vi "StateMachineExecute.vi"(5 "States finished?":bool=TRUE, 8 "error in (no error)":errorcluster, 11 "StateMachine in":refnum<class "StateMachine.lvclass">) -> (0 "error out":errorcluster, 2 "output cluster":T1, 3 "StateMachine out":refnum<class "StateMachine.lvclass">)   [LabVIEW 2018, in "StateMachine.lvclass"]
uses:
  StateMachine.lvclass
  StateMachine.lvclass/StateMachine.ctl
  <vilib>/Rock Robotics/WPI/ThirdParty/Phoenix-LabVIEW/Motor Controller/Controls/CTRE_Phoenix_MotorControl_ControlMode.ctl
  <vilib>/Rock Robotics/WPI/Solenoid/WPI_SolenoidSetEnum.vi
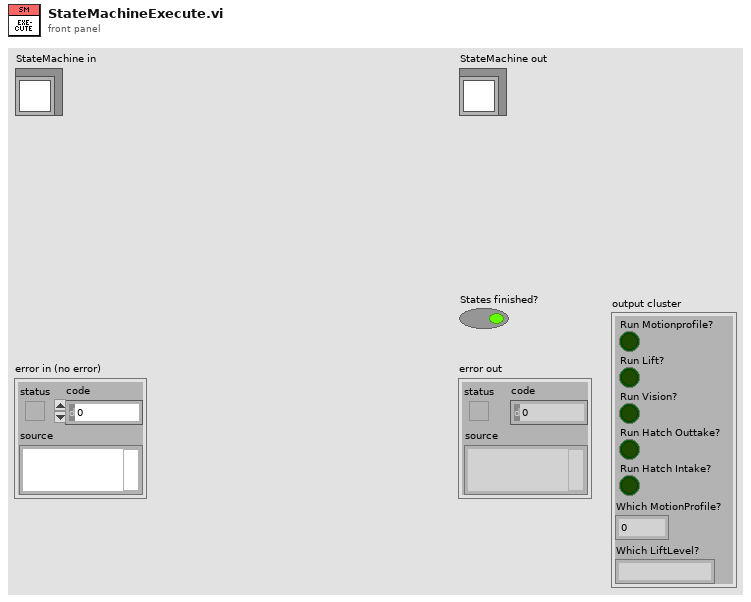
[diagram p1: front panel]
types:
  T1 = cluster{"Run Motionprofile?":bool, "Run Lift?":bool, "Run Vision?":bool, "Run Hatch Outtake?":bool, "Run Hatch Intake?":bool, "Which LiftLevel?":string, "Which MotionProfile?":dbl}
  T2 = cluster{"Run Motionprofile?":bool, "Run Lift?":bool, "Run Vision?":bool, "Run Hatch Outtake?":bool, "Run Hatch Intake?":bool, "Which LiftLevel?":string, "Which MotionProfile?":i32}
  T3 = typedef "CTRE_Phoenix_MotorControl_ControlMode.ctl" = u16
  T4 = typedef "WPI_MotorControlDeviceRef.ctl" = cluster{"DeviceStatus":errorcluster, "Type":T5, "PWM":cluster{"PWM Channel":T6, "DeadBand":T7}, "CAN":cluster{"Device Number":u8, "SetOutput VI Ref":variant, "GetOutput VI Ref":variant, "Enable VI Ref":variant, "Disable VI Ref":variant, "Data":variant}, "Invert":bool, "DIO PWM":cluster{"PWM \"Enable\" Channel":T6, "DIOChannel":T8, "PWM Rate":dbl}}
  T5 = typedef "WPI_MotorControlType.ctl" = enum16{"PWM", "CAN", "DIO PWM"}
  T6 = typedef "FPGA_DIOPWMChannel.ctl" = enum8{"PWM 0", "PWM 1", "PWM 2", "PWM 3", "PWM 4", "PWM 5", "PWM 6", "PWM 7", "PWM 8", "PWM 9", "PWM MXP 0", "PWM MXP 1", "PWM MXP 2", "PWM MXP 3", "PWM MXP 4", "PWM MXP 5", "PWM MXP 6", "PWM MXP 7", "PWM MXP 8", "PWM MXP 9", "Invalid"}
  T7 = typedef "WPI_PWMDeadband.ctl" = cluster{"Name":string, "maxPositivePwm":i32, "minPositivePwm":i32, "centerPwm":i32, "maxNegativePwm":i32, "minNegativePwm":i32, "angularRange":u16}
  T8 = typedef "FPGA_DIOChannel.ctl" = enum8{"DIO 0", "DIO 1", "DIO 2", "DIO 3", "DIO 4", "DIO 5", "DIO 6", "DIO 7", "DIO 8", "DIO 9", "DIO MXP 0", "DIO MXP 1", "DIO MXP 2", "DIO MXP 3", "DIO MXP 4", "DIO MXP 5", "DIO MXP 6", "DIO MXP 7", "DIO MXP 8", "DIO MXP 9", "DIO MXP 10", "DIO MXP 11", "DIO MXP 12", "DIO MXP 13", "DIO MXP 14", "DIO MXP 15", "SPI Port CS1", "SPI Port CS2", "SPI Port CS3", "SPI Port MISO", "SPI Port MOSI", "Invalid"}
  T9 = typedef "WPI_SolenoidDevRef.ctl" = cluster{"DevStatus":errorcluster, "Pneumatics Control Module":u8, "Forward Solenoid Channel":T10, "Reverse Solenoid Channel":T10}
  T10 = typedef "WPI_SolenoidChannel.ctl" = enum8{"Solenoid 0", "Solenoid 1", "Solenoid 2", "Solenoid 3", "Solenoid 4", "Solenoid 5", "Solenoid 6", "Solenoid 7", "Invalid"}
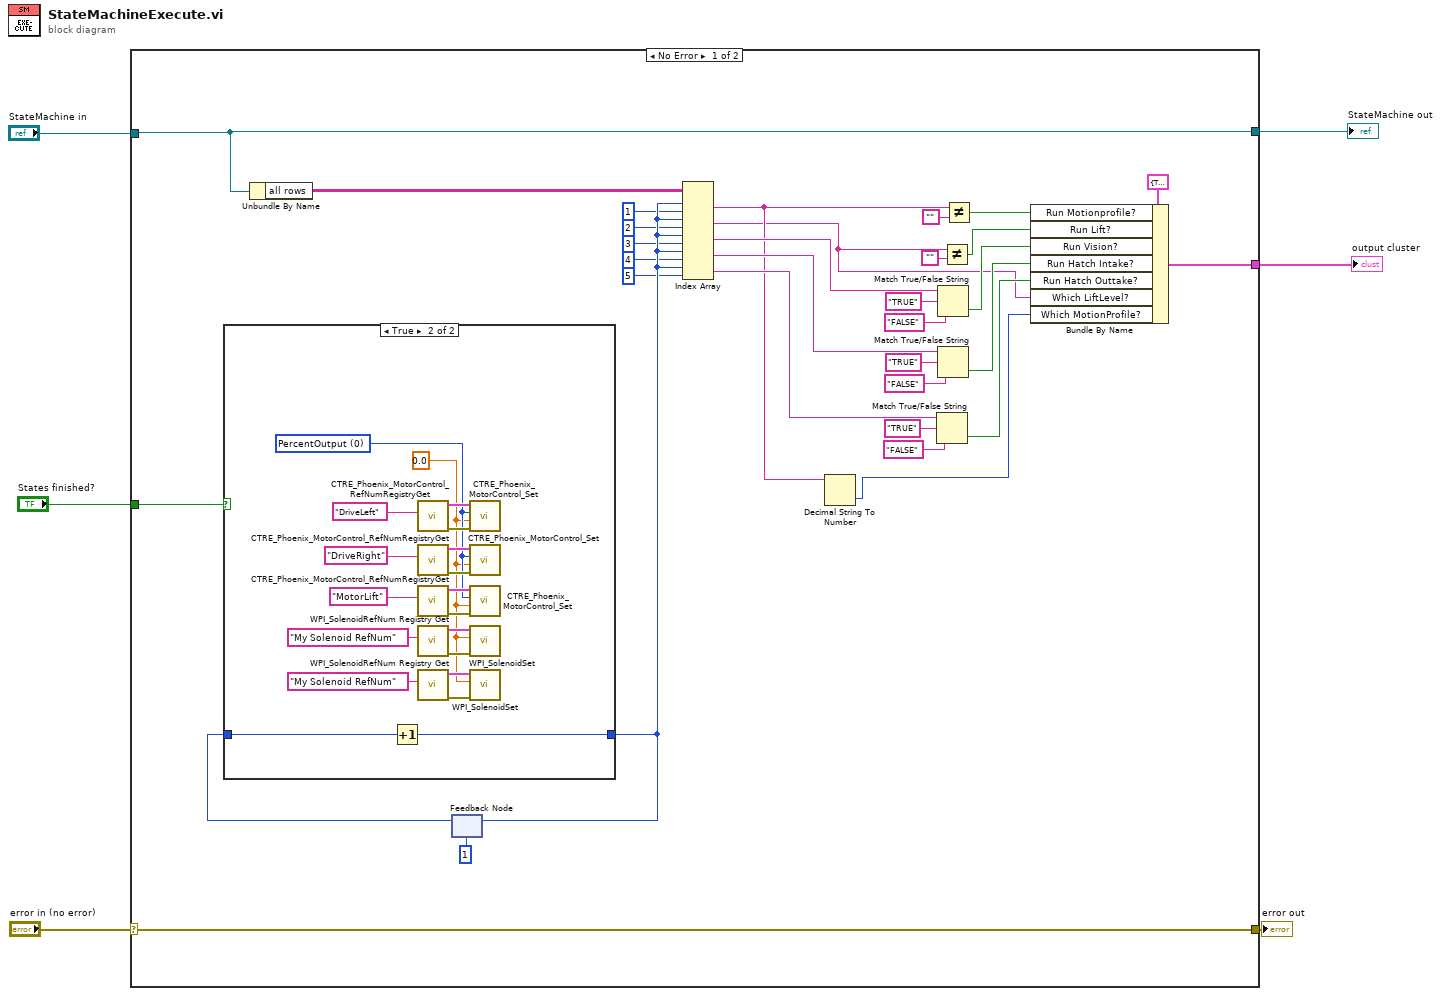
[diagram p0: block diagram]
diagram:
  n1 = case shown="No Error" "error in (no error)" {
    selector: "error in (no error)" -> [w39 w61]
    tunnel: [w39 w61] -> w5
    tunnel: [w11 w60] -> w3
    tunnel: "StateMachine in" -> [w11 w60]
    tunnel: [w12 _] -> w2
    tunnel: "States finished?" -> [w7 _]
    frame No Error {
      n2 = Unbundle By Name(w11) -> ("all rows"=w38:string[][])
      n3 = feedback #1(1) -> (w37:i32)
      n4 = case shown="True" w7 {
        tunnel: w37 -> [w40 w42]
        tunnel: [w40 w41] -> w35
        frame False {
        }
        frame True {
          w43 = 0.0 ("Output")
          w44 = T3 0 items=["PercentOutput"=0, "Position"=1, "Velocity"=2, "Current"=3, "Follower"=5, "MotionProfile"=6, "MotionMagic"=7, "MotionProfileArc"=10, "Disabled"=15] ("Control Mode")
          n5 = Increment(x=w42) -> (x+1=w41:i32)
          n6 = call <vilib>:"CTRE_Phoenix_MotorControl_RefNumRegistryGet.vi"("refnum name"="DriveLeft") -> ("error out"=w59:errorcluster, "PhoenixMotorControlDevRef"=w58:T4)  [unwired: 9 in]
          n7 = call <vilib>:"CTRE_Phoenix_MotorControl_RefNumRegistryGet.vi"("refnum name"="DriveRight") -> ("error out"=w56:errorcluster, "PhoenixMotorControlDevRef"=w55:T4)  [unwired: 9 in]
          n8 = call <vilib>:"CTRE_Phoenix_MotorControl_RefNumRegistryGet.vi"("refnum name"="MotorLift") -> ("error out"=w53:errorcluster, "PhoenixMotorControlDevRef"=w52:T4)  [unwired: 9 in]
          n9 = call <vilib>:"WPI_SolenoidRefNum Registry Get.vi"("refnum name"="My Solenoid RefNum") -> ("error out"=w50:errorcluster, "SolenoidDevRef"=w49:T9)  [unwired: 9 in]
          n10 = call <vilib>:"WPI_SolenoidRefNum Registry Get.vi"("refnum name"="My Solenoid RefNum") -> ("error out"=w47:errorcluster, "SolenoidDevRef"=w46:T9)  [unwired: 9 in]
          n11 = call <vilib>:"CTRE_Phoenix_MotorControl_Set.vi"("error in (no error)"=w59, "Output"=w43, "Control Mode"=w44, "PhoenixMotorControlDevRef"=w58) -> ()  [unwired: 6 in, 2 out]
          n12 = call <vilib>:"CTRE_Phoenix_MotorControl_Set.vi"("error in (no error)"=w56, "Output"=w43, "Control Mode"=w44, "PhoenixMotorControlDevRef"=w55) -> ()  [unwired: 6 in, 2 out]
          n13 = call <vilib>:"CTRE_Phoenix_MotorControl_Set.vi"("error in (no error)"=w53, "Output"=w43, "Control Mode"=w44, "PhoenixMotorControlDevRef"=w52) -> ()  [unwired: 6 in, 2 out]
          n14 = call-poly <vilib>:"WPI_SolenoidSet.vi"("error in (no error)"=w50, "Value"=w43, "SolenoidDevRef"=w49) -> ()  [unwired: 7 in, 2 out]
          n15 = call-poly <vilib>:"WPI_SolenoidSet.vi"("error in (no error)"=w47, "Value"=w43, "SolenoidDevRef"=w46) -> ()  [unwired: 7 in, 2 out]
        }
      }
      n16 = feedback-in #1(w35) -> ()
      n17 = Index Array(array=w38, index (row) #1=w35, index (col) #1=1 ("disabled index (col)"), index (row) #2=w35, index (col) #2=2 ("disabled index (col)"), index (row) #3=w35, index (col) #3=3 ("disabled index (col)"), index (row) #4=w35, index (col) #4=4 ("disabled index (col)"), index (row) #5=w35, index (col) #5=5 ("disabled index (col)")) -> (element #1=w10:string, element #2=w8:string, element #3=w29:string, element #4=w22:string, element #5=w21:string)
      n18 = Decimal String To Number(string=w10) -> (number=w9:i32)  [unwired: 2 in, 1 out]
      n19 = Match True/False String(2:"FALSE" ("false string"), 3:"TRUE" ("true string"), 4:w21) -> (0:w13:bool)  [unwired: 1 out]
      n20 = Match True/False String(2:"FALSE" ("false string"), 3:"TRUE" ("true string"), 4:w29) -> (0:w15:bool)  [unwired: 1 out]
      n21 = Match True/False String(2:"FALSE" ("false string"), 3:"TRUE" ("true string"), 4:w22) -> (0:w14:bool)  [unwired: 1 out]
      n22 = Not Equal?(x=w8, y="") -> (x != y?=w16:bool)
      n23 = Not Equal?(x=w10, y="") -> (x != y?=w17:bool)
      n24 = Bundle By Name(cluster=T2 {"Run Motionprofile?"=TRUE, "Run Lift?"=TRUE, "Run Vision?"=TRUE, "Run Hatch Outtake?"=TRUE, "Run Hatch Intake?"=TRUE, "Which LiftLevel?"="", "Which MotionProfile?"=0}, "Run Motionprofile?"=w17, "Run Lift?"=w16, "Run Vision?"=w15, "Run Hatch Intake?"=w14, "Run Hatch Outtake?"=w13, "Which LiftLevel?"=w8, "Which MotionProfile?"=w9) -> (w12:T2)
    }
    frame Error {
    }
  }
  "error out" <- w5
  "StateMachine out" <- w3
  "output cluster" <- w2
